vi "Decorator.vi"(8 "error in (no error)":errorcluster, 10 "DecoratorData in":refnum<class "Data.lvclass">, 11 "DataVer1 in":refnum<class "DataVer1.lvclass">) -> (0 "error out":errorcluster, 3 "DataVer1 out":refnum<class "DataVer1.lvclass">)   [LabVIEW 2013, in "DataVer1.lvclass"]
uses:
  DataVer1.lvclass
  Data.lvclass/Data.lvclass
  DataVer1.lvclass/DataVer1.ctl
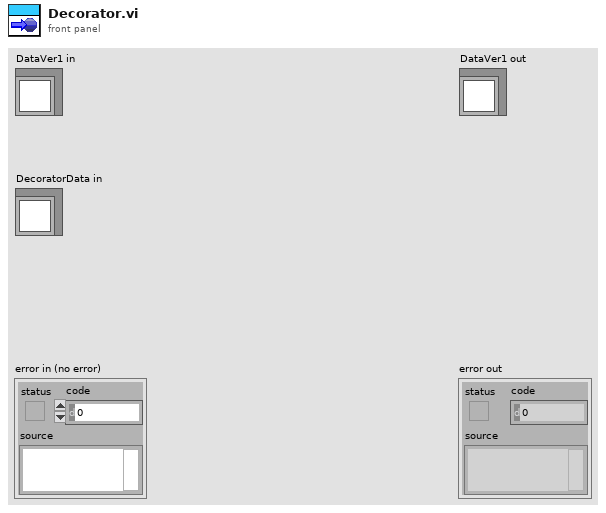
[diagram p1: front panel]
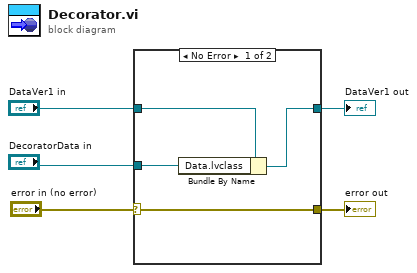
[diagram p0: block diagram]
diagram:
  n1 = case shown="No Error" "error in (no error)" {
    selector: "error in (no error)" -> [w9 w11]
    tunnel: [w9 w11] -> w1
    tunnel: [w6 w10] -> w4
    tunnel: "DataVer1 in" -> [w7 w10]
    tunnel: "DecoratorData in" -> [w8 _]
    frame No Error {
      n2 = Bundle By Name(cluster=w7, "Data.lvclass"=w8) -> (w6:refnum<class "DataVer1.lvclass">)
    }
    frame Error {
    }
  }
  "error out" <- w1
  "DataVer1 out" <- w4
